vi "Wait (ms).vi"(1 "Execute":bool=TRUE, 2 "milliseconds to wait":u32) -> (4 "Done Executing":bool)   [LabVIEW 2011]
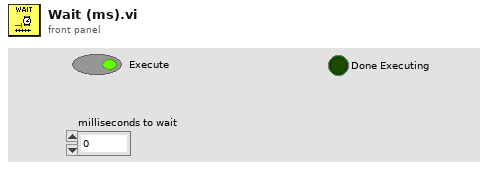
[diagram p1: front panel]
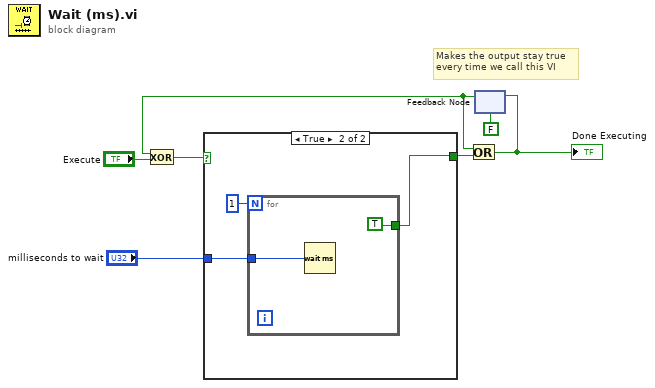
[diagram p0: block diagram]
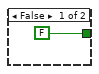
[diagram p2: hidden frame]
diagram:
  # "Makes the output stay true\nevery time we call this VI"
  n1 = feedback #1(FALSE) -> (w3:bool)
  n2 = Exclusive Or(1:"Execute", 2:w3) -> (0:w7:bool)
  n3 = case shown="True" w7 {
    tunnel: [FALSE w10] -> w5
    tunnel: "milliseconds to wait" -> [_ w9]
    frame False {
    }
    frame True {
      n4 = for {
        N: 1 -> [_]
        tunnel: [TRUE] -> w10
        tunnel: w9 -> [w12]
        n5 = Wait (ms)(milliseconds to wait=w12) -> ()  [unwired: 1 out]
      }
    }
  }
  n6 = Or(x=w3, y=w5) -> (x .or. y?=w2:bool)
  "Done Executing" <- w2
  n7 = feedback-in #1(w2) -> ()
